vi "Sample Pad Example (Arduino Controller).vi"() -> ()   [LabVIEW 2020]
doc: "A simple sample pad, which can trigger up to 16 simultaneous sound effects. Demonstrates the Mixer component, including file loading, playback, and mixer audio monitoring via a music visualizer."
uses:
  Mixer/Channel/Controls/Channel State.ctl
  Mixer/Mixer/Mixer.lvclass/Mixer.ctl
  <vilib>/MakerHub/LINX/Public/Peripherals/Digital/Digital Read N Chans.vi
  e8fa8eb6-c38c-4b8a-b362-922d187964a0.vi
  <vilib>/MakerHub/LINX/Private/Local IO/LinxDigitalRead.vi
  <vilib>/MakerHub/LINX/Public/Utilities/Check Channel.vi
  <vilib>/MakerHub/LINX/Public/Utilities/Open Serial.vi
  <vilib>/MakerHub/LINX/Private/Utilties/Generate Error.vi
  Mixer/Mixer/Polymorphic VIs/Channel Load (Path).vi
  Mixer/Mixer/Mixer.lvclass
  Mixer/Channel/Channel.lvclass
  <vilib>/MakerHub/LINX/LMH-LINX.lvlib
panel:
  in  "Serial Port":refnum<visa-resource-name>="COM11"
  in  "Visualizer":bool
  in  "Sample Path":path
  in  "Stop":bool
  in  "Play 4":bool caption="V"
  in  "Play 3":bool caption="C"
  in  "Play 2":bool caption="X"
  in  "Play 1":bool caption="Z"
  in  "Play 8":bool caption="F"
  in  "Play 7":bool caption="D"
  in  "Play 6":bool caption="S"
  in  "Play 5":bool caption="A"
  in  "Play 12":bool caption="R"
  in  "Play 11":bool caption="E"
  in  "Play 10":bool caption="W"
  in  "Play 9":bool caption="Q"
  in  "Play 16":bool caption="4"
  in  "Play 15":bool caption="3"
  in  "Play 14":bool caption="2"
  in  "Play 13":bool caption="1"
  # "Multi-channel Mixer Demo"
  # "G"
  # "-Audio"
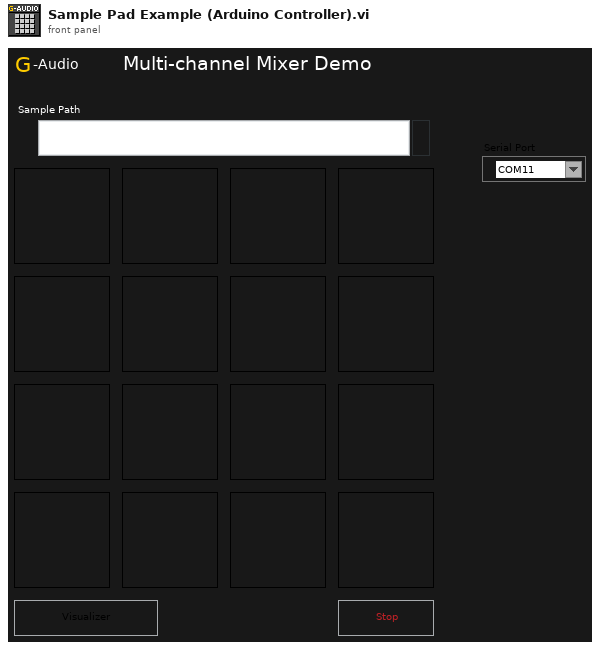
[diagram p1: front panel]
types:
  T1 = typedef "G-Audio.lvlib/Channel.lvclass/Channel State.ctl" = enum16{"Empty", "Error", "Loading", "Loaded", "Stopped", "Paused", "Playing", "Retrigger"}
  T2 = typedef "LMH-LINX.lvlib/LINX Ref.ctl" = cluster{"IO":T3, "Interface":T4, "LINX Device Config":T5}
  T3 = typedef "LMH-LINX.lvlib/Platform.ctl" = enum16{"Remote", "Local"}
  T4 = typedef "LMH-LINX.lvlib/Interface.ctl" = enum16{"Serial", "TCP"}
  T5 = typedef "LMH-LINX.lvlib/Device.lvlib/LINX Device Config.ctl" = cluster{"Interface":T4, "COM Port":refnum<visa-resource-name>, "TCP Configuration":T6, "Device Family":u8, "Device ID":u8, "Device Name":string, "TCP Ref":refnum<k5>, "Channels":T7}
  T6 = typedef "LMH-LINX.lvlib/Device.lvlib/TCP Config.ctl" = cluster{"IP Address":string, "Port":u16}
  T7 = typedef "LMH-LINX.lvlib/Channels.ctl" = cluster{"DI":u8[], "DO":u8[], "AI":u8[], "AO":u8[], "PWM":u8[], "QE":u8[], "UART":u8[], "I2C 2":u8[], "SPI":u8[], "CAN":u8[], "Servo":u8[], "AI Ref (V)":dbl, "AI Resolution (Bits)":u8, "AO Ref (V)":dbl, "AO Resolution (Bits)":u8}
  T8 = enum32{"Invalid", "Standard", "Closed", "Hidden", "Minimized", "Maximized"}
  T9 = typedef "G-Audio.lvlib/Channel.lvclass/Channel Status.ctl" = cluster{"Frame":u64, "State":T1, "Volume":dbl}
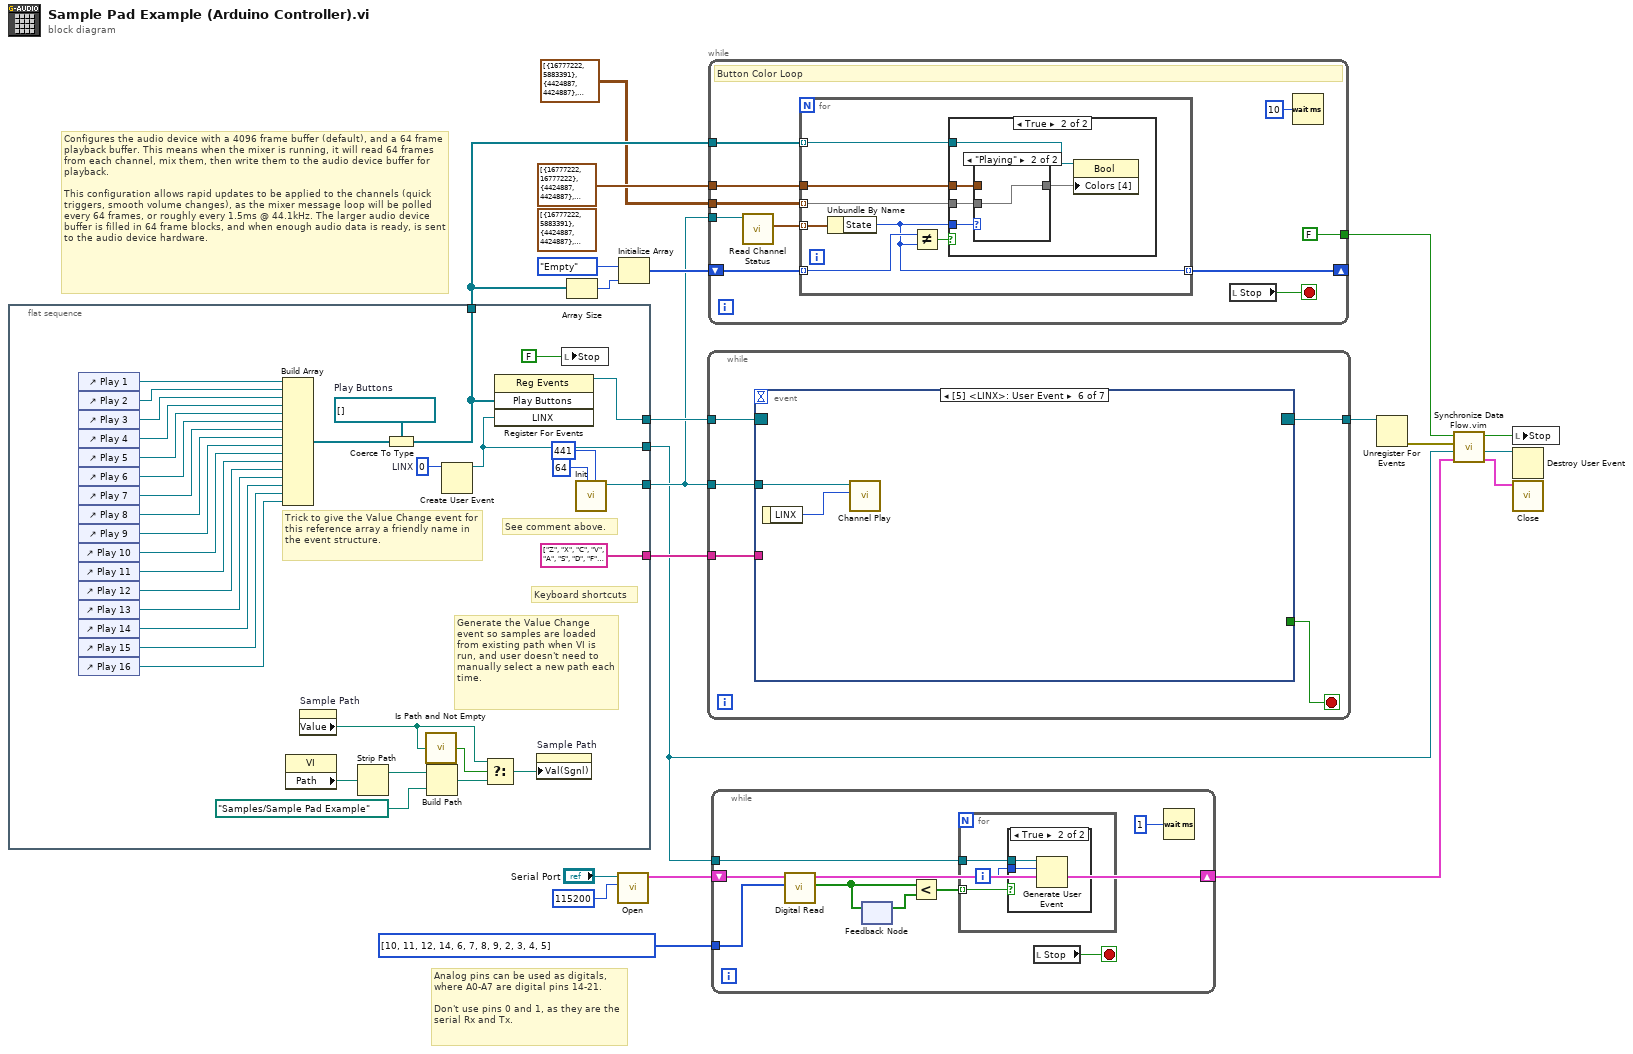
[diagram p0: block diagram]
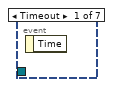
[diagram p5: hidden frame]
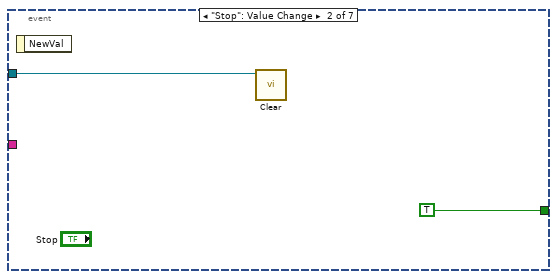
[diagram p6: hidden frame]
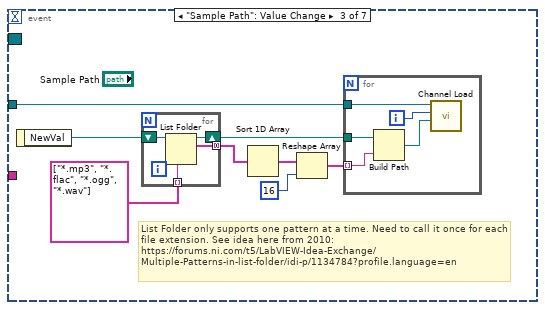
[diagram p7: hidden frame]
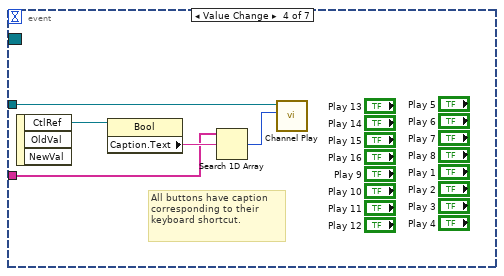
[diagram p8: hidden frame]
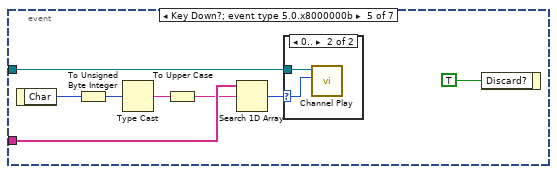
[diagram p9: hidden frame]
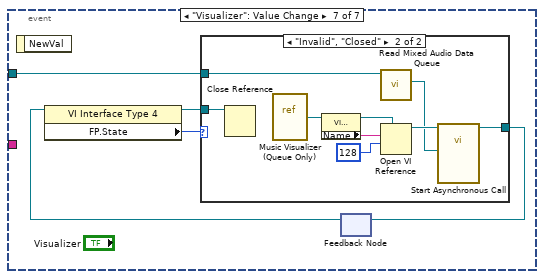
[diagram p11: hidden frame]
diagram:
  (unwired) cluster{"Color Box":u32, "Color Box":u32}[][] [[{"Color Box"=16777222, "Color Box"=5883391}, {"Color Box"=4424887, "Color Box"=4424887}, {"Color Box"=4424887, "Color Box"=4424887}, {"Color Box"=4424887, "Color Box"=4424887}], [{"Color Box"=16777222, "Color Box"=5883391}, {"Color Box"=4424887, "Color Box"=4424887}, {"Color Box"=4424887, "Color Box"=4424887}, {"Color Box"=4424887, "Color Box"=4424887}], [{"Color Box"=16777222, "Color Box"=5883391}, {"Color Box"=4424887, "Color Box"=4424887}, {"Color Box"=4424887, "Color Box"=4424887}, {"Color Box"=4424887, "Color Box"=4424887}], [{"Color Box"=16777222, "Color Box"=5883391}, {"Color Box"=4424887, "Color Box"=4424887}, {"Color Box"=4424887, "Color Box"=4424887}, {"Color Box"=4424887, "Color Box"=4424887}], [{"Color Box"=16777222, "Color Box"=6618880}, {"Color Box"=4424887, "Color Box"=4424887}, {"Color Box"=4424887, "Color Box"=4424887}, {"Color Box"=4424887, "Color Box"=4424887}], [{"Color Box"=16777222, "Color Box"=6618880}, {"Color Box"=4424887, "Color Box"=4424887}, {"Color Box"=4424887, "Color Box"=4424887}, {"Color Box"=4424887, "Color Box"=4424887}], [{"Color Box"=16777222, "Color Box"=6618880}, {"Color Box"=4424887, "Color Box"=4424887}, {"Color Box"=4424887, "Color Box"=4424887}, {"Color Box"=4424887, "Color Box"=4424887}], [{"Color Box"=16777222, "Color Box"=6618880}, {"Color Box"=4424887, "Color Box"=4424887}, {"Color Box"=4424887, "Color Box"=4424887}, {"Color Box"=4424887, "Color Box"=4424887}], [{"Color Box"=16777222, "Color Box"=16746514}, {"Color Box"=4424887, "Color Box"=4424887}, {"Color Box"=4424887, "Color Box"=4424887}, {"Color Box"=4424887, "Color Box"=4424887}], [{"Color Box"=16777222, "Color Box"=16746514}, {"Color Box"=4424887, "Color Box"=4424887}, {"Color Box"=4424887, "Color Box"=4424887}, {"Color Box"=4424887, "Color Box"=4424887}], [{"Color Box"=16777222, "Color Box"=16746514}, {"Color Box"=4424887, "Color Box"=4424887}, {"Color Box"=4424887, "Color Box"=4424887}, {"Color Box"=4424887, "Color Box"=4424887}], [{"Color Box"=16777222, "Color Box"=16746514}, {"Color Box"=4424887, "Color Box"=4424887}, {"Color Box"=4424887, "Color Box"=4424887}, {"Color Box"=4424887, "Color Box"=4424887}], [{"Color Box"=16777222, "Color Box"=16711680}, {"Color Box"=4424887, "Color Box"=4424887}, {"Color Box"=4424887, "Color Box"=4424887}, {"Color Box"=4424887, "Color Box"=4424887}], [{"Color Box"=16777222, "Color Box"=16711680}, {"Color Box"=4424887, "Color Box"=4424887}, {"Color Box"=4424887, "Color Box"=4424887}, {"Color Box"=4424887, "Color Box"=4424887}], [{"Color Box"=16777222, "Color Box"=16711680}, {"Color Box"=4424887, "Color Box"=4424887}, {"Color Box"=4424887, "Color Box"=4424887}, {"Color Box"=4424887, "Color Box"=4424887}], [{"Color Box"=16777222, "Color Box"=16711680}, {"Color Box"=4424887, "Color Box"=4424887}, {"Color Box"=4424887, "Color Box"=4424887}, {"Color Box"=4424887, "Color Box"=4424887}]] ("appended array")
  # "Analog pins can be used as digitals, where A0-A7 are digital pins 14-21.\n\nDon't use pins 0 and 1, as they are the serial Rx and Tx."
  # "Configures the audio device with a 4096 frame buffer (default), and a 64 frame playback buffer. This means when the mixer is running, it will read 64 frames from each channel, mix them, then write them to the audio device buffer for playback.\n\nThis configuration allows rapid updates to be applied to the channels (quick triggers, smooth volume changes), as the mixer message loop will be polled every 64 frames, or roughly every 1.5ms @ 44.1kHz. The larger audio device buffer is filled in 64 frame blocks, and when enough audio data is ready, is sent to the audio device hardware."
  n1 = flat-sequence {
    tunnel: [w54] -> w20
    tunnel: [string[] ["Z", "X", "C", "V", "A", "S", "D", "F", "Q", "W", "E", "R", "1", "2", "3", "4"]] -> w19
    tunnel: [w25] -> w11
    tunnel: [w52] -> w14
    tunnel: [w23] -> w4
    frame #0 {
      w24 = 0  # LINX
      w55 = refnum<vi>[] []  # Play Buttons
      # "Trick to give the Value Change event for this reference array a friendly name in the event structure."
      # "See comment above."
      # "Generate the Value Change event so samples are loaded from existing path when VI is run, and user doesn't need to manually select a new path each time."
      # "Keyboard shortcuts"
      n2 = control-ref of="Play 1"() -> (w49:refnum<vi>)
      n3 = control-ref of="Play 2"() -> (w48:refnum<vi>)
      n4 = control-ref of="Play 3"() -> (w47:refnum<vi>)
      n5 = control-ref of="Play 4"() -> (w46:refnum<vi>)
      n6 = control-ref of="Play 5"() -> (w45:refnum<vi>)
      n7 = control-ref of="Play 6"() -> (w44:refnum<vi>)
      n8 = control-ref of="Play 7"() -> (w43:refnum<vi>)
      n9 = control-ref of="Play 8"() -> (w42:refnum<vi>)
      n10 = control-ref of="Play 9"() -> (w41:refnum<vi>)
      n11 = control-ref of="Play 10"() -> (w40:refnum<vi>)
      n12 = control-ref of="Play 11"() -> (w39:refnum<vi>)
      n13 = control-ref of="Play 12"() -> (w38:refnum<vi>)
      n14 = control-ref of="Play 13"() -> (w37:refnum<vi>)
      n15 = control-ref of="Play 14"() -> (w36:refnum<vi>)
      n16 = control-ref of="Play 15"() -> (w35:refnum<vi>)
      n17 = control-ref of="Play 16"() -> (w34:refnum<vi>)
      n18 = Build Array(w49, w48, w47, w46, w45, w44, w43, w42, w41, w40, w39, w38, w37, w36, w35, w34) -> (w50:refnum<vi>[])
      n19 = property class="VI"() -> ("Path"=w31:path)  [unwired: 2 in, 2 out]
      n20 = property on="Sample Path" class="Path"() -> ("Value"=w27:path)  [unwired: 2 in, 2 out]
      n21 = Strip Path(path=w31) -> (stripped path=w30:path)  [unwired: 1 out]
      n22 = Coerce To Type(0:w50, 1:w55) -> (2:w25:refnum<vi>[])
      n23 = call <vilib>:"Is Path and Not Empty.vi"("path"=w27) -> ("Is Path and Not Empty?"=w33:bool)  [unwired: 4 in]
      n24 = Build Path(base path=w30, name or relative path=path "Samples/Sample Pad Example") -> (appended path=w28:path)
      n25 = Create User Event(user event datatype=w24) -> (user event=w23:refnum<user-event>)  [unwired: 1 in, 1 out]
      n26 = Select(t=w27, s=w33, f=w28) -> (s? t:f=w32:path)
      n27 = register-events(w25, w23) -> (reference out=w54:refnum<event-registration>)  [unwired: 2 in, 1 out]
      n28 = property on="Sample Path" class="Path"("Val(Sgnl)"=w32) -> ()  [unwired: 2 in, 2 out]
      n29 = local write "Stop"(FALSE ("Stop")) -> ()
      n30 = call "Init.vi"("Buffer Size (4096)"=441, "Playback Size (4096)"=64) -> ("Mixer out"=w52:refnum<class "Mixer.lvclass">)  [unwired: 8 in, 1 out]
    }
  }
  n31 = Array Size(array=w11) -> (size(s)=w12:i32)
  n32 = call-poly <vilib>:"Open.vi"("Baud Rate Override"=u32 115200, "Serial Port"="Serial Port") -> ("LINX Resource"=w10:T2)  [unwired: 7 in, 2 out]
  n33 = Initialize Array(Channel_State."Empty" ("State"), w12) -> (w21:T1[])
  n34 = while {
    tunnel: w20 -> [w60]
    tunnel: w14 -> [w59]
    tunnel: w19 -> [w58]
    tunnel: [w56] -> w18
    stop <- w57 stop-if-true
    n35 = event shown="[5] <LINX>: User Event" {
      selector: w60 -> [_ _ _ _ _ _ _]
      dyn-events: [_ _ _ _ _ _ _] -> w56
      timeout: _ -> [_ _ _ _ _ _ _]
      tunnel: w59 -> [_ w62 w68 w83 w92 w96 w100]
      tunnel: w58 -> [_ _ _ w81 w90 _ _]
      tunnel: [_ TRUE _ _ _ _ _] -> w57
      event Timeout {
        n36 = event-data() -> ()  [unwired: 1 in, 1 out]
      }
      event "Stop": Value Change {
        n37 = event-data() -> ()  [unwired: 1 in, 1 out]
        n38 = call "Clear.vi"("Mixer in"=w62) -> ()  [unwired: 10 in, 1 out]
      }
      event "Sample Path": Value Change {
        # "List Folder only supports one pattern at a time. Need to call it once for each file extension. See idea here from 2010:\nhttps://forums.ni.com/t5/LabVIEW-Idea-Exchange/Multiple-Patterns-in-list-folder/idi-p/1134784?profile.language=en"
        n39 = event-data() -> ("NewVal"=w63:path)  [unwired: 1 in]
        n40 = for {
          shift-right: [w74] -> w69
          shift-left: w63 -> [w73]
          tunnel: string[] ["*.mp3", "*.flac", "*.ogg", "*.wav"] -> [w72] mode=indexing
          tunnel: [w71] -> w65 mode=concatenating
          n41 = List Folder(path=w73, pattern=w72) -> (path out=w74:path, filenames=w71:string[])  [unwired: 2 in, 2 out]
        }
        n42 = Sort 1D Array(array=w65) -> (sorted array=w64:string[])
        n43 = Reshape Array(w64, 16 ("dimension size")) -> (w70:string[])
        n44 = for {
          tunnel: w70 -> [w79] mode=indexing
          tunnel: w69 -> [w78]
          tunnel: w68 -> [w77]
          i -> [w76]
          n45 = Build Path(base path=w78, name or relative path=w79) -> (appended path=w75:path)
          n46 = call-poly "Channel Load.vi"("Path"=w75, "Channel Index"=w76, "Mixer in"=w77) -> ()  [unwired: 7 in, 2 out]
        }
      }
      event Value Change {
        # "All buttons have caption corresponding to their keyboard shortcut."
        n47 = event-data() -> ("CtlRef"=w84:refnum<vi>)  [unwired: 1 in, 2 out]
        n48 = property class="Bool"(reference=w84) -> ("Caption.Text"=w82:string)  [unwired: 1 in, 2 out]
        n49 = Search 1D Array(1D array=w81, element=w82) -> (index of element=w80:i32)  [unwired: 1 in]
        n50 = call "Channel Play.vi"("Channel Index"=w80, "Mixer in"=w83) -> ()  [unwired: 8 in, 2 out]
      }
      event Key Down?; event type 5.0.x8000000b {
        n51 = event-data() -> ("Char"=w91:i16)  [unwired: 1 in]
        n52 = To Unsigned Byte Integer(number=w91) -> (unsigned 8bit integer=w87:u8)
        n53 = Type Cast(x=w87) -> (*(type *) &x=w85:string)  [unwired: 1 in]
        n54 = To Upper Case(1:w85) -> (0:w88:string)
        n55 = Search 1D Array(1D array=w90, element=w88) -> (index of element=w86:i32)  [unwired: 1 in]
        n56 = case shown="0.." w86 {
          selector: w86 -> [_ w93]
          tunnel: w92 -> [_ w94]
          frame Default {
          }
          frame 0.. {
            n57 = call "Channel Play.vi"("Channel Index"=w93, "Mixer in"=w94) -> ()  [unwired: 8 in, 2 out]
          }
        }
        n58 = event-data("Discard?"=TRUE) -> ()  [unwired: 1 in, 1 out]
      }
      event User Event {
        n59 = event-data() -> ("LINX"=w95:i32)  [unwired: 1 in]
        n60 = call "Channel Play.vi"("Channel Index"=w95, "Mixer in"=w96) -> ()  [unwired: 8 in, 2 out]
      }
      event "Visualizer": Value Change {
        n61 = event-data() -> ()  [unwired: 1 in, 1 out]
        n62 = feedback #1() -> (w97:refnum<vi>)  [unwired: 1 in]
        n63 = property class="VI Interface Type 4"(reference=w97) -> (reference out=w99:refnum<vi>, "FP.State"=w98:T8)  [unwired: 1 in, 1 out]
        n64 = case shown="\"Invalid\", \"Closed\"" w98 {
          tunnel: [w102 w106] -> w101
          tunnel: w100 -> [_ w105]
          tunnel: w99 -> [w102 w103]
          frame Default {
          }
          frame "Invalid", "Closed" {
            n65 = Close Reference(reference=w103) -> ()  [unwired: 1 in, 1 out]
            n66 = vi-ref "Music Visualizer (Queue Only).vi"() -> (w111:refnum<vi>)
            n67 = property class="VI (strict)"(reference=w111) -> (reference out=w109:refnum<vi>, "Name"=w110:string)  [unwired: 1 in, 1 out]
            n68 = call "Read Mixed Audio Data Queue.vi"("Mixer in"=w105) -> ("Mixed Audio Data"=w104:refnum<queue>)  [unwired: 8 in, 2 out]
            n69 = Open VI Reference(type specifier VI Refnum (for type only)=w109, vi path=w110, options=128) -> (vi reference=w107:refnum<vi>)  [unwired: 3 in, 1 out]
            n70 = call-by-ref "Start Asynchronous Call"(reference=w107, "Mixed Audio Data"=w104) -> (reference out=w106:refnum<vi>)  [unwired: 12 in, 1 out]
          }
        }
        n71 = feedback-in #1(w101) -> ()
      }
    }
  }
  n72 = while {
    tunnel: w14 -> [w121]
    tunnel: w11 -> [w119]
    tunnel: cluster{u32, u32}[] [{16777222, 16777222}, {4424887, 4424887}, {4424887, 4424887}, {4424887, 4424887}] ("Colors [4]") -> [w118]
    tunnel: cluster{"Color Box":u32, "Color Box":u32}[][] [[{"Color Box"=16777222, "Color Box"=5883391}, {"Color Box"=4424887, "Color Box"=4424887}, {"Color Box"=4424887, "Color Box"=4424887}, {"Color Box"=4424887, "Color Box"=4424887}], [{"Color Box"=16777222, "Color Box"=6618880}, {"Color Box"=4424887, "Color Box"=4424887}, {"Color Box"=4424887, "Color Box"=4424887}, {"Color Box"=4424887, "Color Box"=4424887}], [{"Color Box"=16777222, "Color Box"=16746514}, {"Color Box"=4424887, "Color Box"=4424887}, {"Color Box"=4424887, "Color Box"=4424887}, {"Color Box"=4424887, "Color Box"=4424887}], [{"Color Box"=16777222, "Color Box"=16722505}, {"Color Box"=4424887, "Color Box"=4424887}, {"Color Box"=4424887, "Color Box"=4424887}, {"Color Box"=4424887, "Color Box"=4424887}], [{"Color Box"=16777222, "Color Box"=5883391}, {"Color Box"=4424887, "Color Box"=4424887}, {"Color Box"=4424887, "Color Box"=4424887}, {"Color Box"=4424887, "Color Box"=4424887}], [{"Color Box"=16777222, "Color Box"=6618880}, {"Color Box"=4424887, "Color Box"=4424887}, {"Color Box"=4424887, "Color Box"=4424887}, {"Color Box"=4424887, "Color Box"=4424887}], [{"Color Box"=16777222, "Color Box"=16746514}, {"Color Box"=4424887, "Color Box"=4424887}, {"Color Box"=4424887, "Color Box"=4424887}, {"Color Box"=4424887, "Color Box"=4424887}], [{"Color Box"=16777222, "Color Box"=16722505}, {"Color Box"=4424887, "Color Box"=4424887}, {"Color Box"=4424887, "Color Box"=4424887}, {"Color Box"=4424887, "Color Box"=4424887}], [{"Color Box"=16777222, "Color Box"=5883391}, {"Color Box"=4424887, "Color Box"=4424887}, {"Color Box"=4424887, "Color Box"=4424887}, {"Color Box"=4424887, "Color Box"=4424887}], [{"Color Box"=16777222, "Color Box"=6618880}, {"Color Box"=4424887, "Color Box"=4424887}, {"Color Box"=4424887, "Color Box"=4424887}, {"Color Box"=4424887, "Color Box"=4424887}], [{"Color Box"=16777222, "Color Box"=16746514}, {"Color Box"=4424887, "Color Box"=4424887}, {"Color Box"=4424887, "Color Box"=4424887}, {"Color Box"=4424887, "Color Box"=4424887}], [{"Color Box"=16777222, "Color Box"=16722505}, {"Color Box"=4424887, "Color Box"=4424887}, {"Color Box"=4424887, "Color Box"=4424887}, {"Color Box"=4424887, "Color Box"=4424887}], [{"Color Box"=16777222, "Color Box"=5883391}, {"Color Box"=4424887, "Color Box"=4424887}, {"Color Box"=4424887, "Color Box"=4424887}, {"Color Box"=4424887, "Color Box"=4424887}], [{"Color Box"=16777222, "Color Box"=6618880}, {"Color Box"=4424887, "Color Box"=4424887}, {"Color Box"=4424887, "Color Box"=4424887}, {"Color Box"=4424887, "Color Box"=4424887}], [{"Color Box"=16777222, "Color Box"=16746514}, {"Color Box"=4424887, "Color Box"=4424887}, {"Color Box"=4424887, "Color Box"=4424887}, {"Color Box"=4424887, "Color Box"=4424887}], [{"Color Box"=16777222, "Color Box"=16722505}, {"Color Box"=4424887, "Color Box"=4424887}, {"Color Box"=4424887, "Color Box"=4424887}, {"Color Box"=4424887, "Color Box"=4424887}]] ("appended array") -> [w117]
    tunnel: [FALSE ("Stop")] -> w15
    shift-right: [w113] -> _
    shift-left: w21 -> [w112]
    stop <- w115 stop-if-true
    # "Button Color Loop"
    n73 = call "Read Channel Status.vi"("Mixer in"=w121) -> ("Channel Status"=w120:T9[])  [unwired: 8 in, 2 out]
    n74 = for {
      tunnel: w120 -> [w128] mode=indexing
      tunnel: w119 -> [w127] mode=indexing
      tunnel: w118 -> [w126]
      tunnel: w117 -> [w125] mode=indexing
      tunnel: [w122] -> w113 mode=indexing
      tunnel: w112 -> [w124] mode=indexing
      n75 = Unbundle By Name(w128) -> ("State"=w122:T1)
      n76 = Not Equal?(x=w124, y=w122) -> (x != y?=w123:bool)
      n77 = case shown="True" w123 {
        tunnel: w127 -> [_ w133]
        tunnel: w126 -> [_ w132]
        tunnel: w125 -> [_ w130]
        tunnel: w122 -> [_ w129]
        frame False {
        }
        frame True {
          n78 = case shown="\"Playing\"" w129 {
            tunnel: w132 -> [w134 _]
            tunnel: [w134 w135] -> w131
            tunnel: w130 -> [_ w135]
            frame Default {
            }
            frame "Playing" {
            }
          }
          n79 = property class="Bool"(reference=w133, "Colors [4]"=w131) -> ()  [unwired: 1 in, 2 out]
        }
      }
    }
    n80 = local read "Stop"() -> (w115:bool)
    n81 = Wait (ms)(milliseconds to wait=u32 10) -> ()  [unwired: 1 out]
  }
  n82 = while {
    tunnel: u8[] [10, 11, 12, 14, 6, 7, 8, 9, 2, 3, 4, 5] -> [w143]
    tunnel: w4 -> [w139]
    shift-right: [w138] -> w6
    shift-left: w10 -> [w144]
    stop <- w137 stop-if-true
    n83 = call-poly <vilib>:"Digital Read.vi"("DI Channels"=w143, "LINX Resource"=w144) -> ("Values"=w142:bool[], "LINX Resource"=w138:T2)  [unwired: 7 in, 1 out]
    n84 = feedback-in #2(w142) -> ()
    n85 = feedback #2() -> (w141:bool[])  [unwired: 1 in]
    n86 = Less?(x=w142, y=w141) -> (x < y?=w140:bool[])
    n87 = for {
      tunnel: w140 -> [w146] mode=indexing
      tunnel: w139 -> [w147]
      i -> [w145]
      n88 = case shown="True" w146 {
        tunnel: w147 -> [_ w149]
        tunnel: w145 -> [_ w148]
        frame False {
        }
        frame True {
          n89 = Generate User Event(user event=w149, event data cluster=w148) -> ()  [unwired: 2 in, 2 out]
        }
      }
    }
    n90 = local read "Stop"() -> (w137:bool)
    n91 = Wait (ms)(milliseconds to wait=u32 1) -> ()  [unwired: 1 out]
  }
  n92 = Unregister For Events(event registration refnum=w18) -> (error out=w7:errorcluster)  [unwired: 1 in]
  n93 = call "Synchronize Data Flow.vim"("input 4"=w6, "input 3"=w4, "input 2"=w7, "input 1"=w15) -> ("output 4"=w5:T2, "output 3"=w3:refnum<user-event>, "output 1"=w16:bool)  [unwired: 1 out]
  n94 = local write "Stop"(w16) -> ()
  n95 = Destroy User Event(user event=w3) -> ()  [unwired: 1 in, 1 out]
  n96 = call <vilib>:"Close.vi"("LINX Resource"=w5) -> ()  [unwired: 10 in, 1 out]
